vi "Draw.vi"(8 "error in (no error)":errorcluster, 10 "picture in (empty picture)":picture, 11 "Empty in":refnum<class "Empty.lvclass">) -> (0 "error out":errorcluster, 2 "picture out":picture, 3 "Empty out":refnum<class "Empty.lvclass">)   [LabVIEW 2018, in "Empty.lvclass"]
doc: "Draw an empty graphics object. Does nothing."
uses:
  Empty.lvclass
panel:
  # "expressionflow.com"
  # "Copyright (c) 2008 Tomi Maila. All rights reserved."
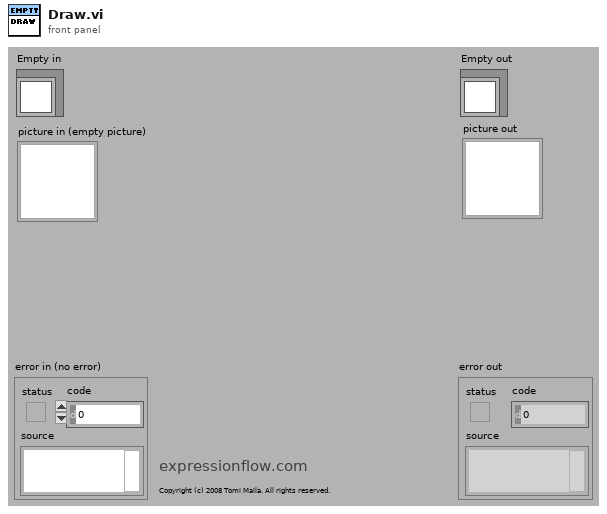
[diagram p1: front panel]
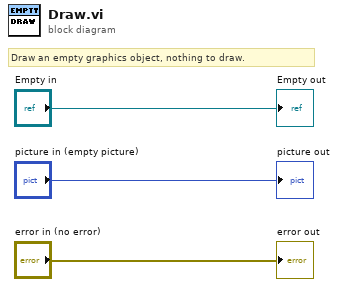
[diagram p0: block diagram]
diagram:
  # "Draw an empty graphics object, nothing to draw."
  "error out" <- "error in (no error)"
  "Empty out" <- "Empty in"
  "picture out" <- "picture in (empty picture)"
